vi "校准中 (子VI).vi"(0 "曲线模型":refnum<vi>, 1 "校准按钮":refnum<vi>) -> ()   [LabVIEW 2016, in "斯坦道氨氮.lvlib"]
uses:
  <vilib>/ptbypt/NI_PtbyPt.lvlib
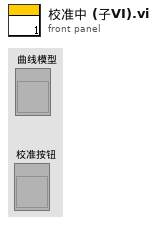
[diagram p1: front panel]
types:
  T1 = enum8{"Enabled", "Disabled", "Disabled and Grayed Out"}
  T2 = cluster{"时间标识":timestamp, "设备":string, "日志信息":string, "流程参数":string}
  T3 = cluster{"系统时间":timestamp, "工作状态":enum16{"空闲", "水样测试", "标样核查", "零点核查", "跨度核查", "空白测试", "平行样测试", "加标回收", "空白校准", "标样校准", "初始化（清洗）"}, "测量模式":enum16{"待机", "连续模式", "周期模式", "定点模式", "受控模式", "手动模式"}, "告警代码":u16, "故障代码":u16, "日志代码":u16, "软件版本":u16, "F0":sgl, "F1":sgl, "F2":sgl, "F3":sgl, "T":sgl, "H":sgl, "id":u16, "flowid":u16, "量程":u16, "总磷控温温度1":sgl, "营养盐控温温度2":sgl, "ADC":sgl}
  T4 = enum16{"空闲", "水样测试", "标样核查", "零点核查", "跨度核查", "空白测试", "平行样测试", "加标回收", "空白校准", "标样校准", "初始化（清洗）"}
  T5 = cluster{"因子编码":u32, "单位":u16, "标样参考值":sgl, "水样数据时间":timestamp, "水样实测值":sgl, "水样数据标识":string, "标样数据时间":timestamp, "标样实测值":sgl, "标样数据标识":string, "空白数据时间":timestamp, "空白实测值":sgl, "空白数据标识":string, "零点核查数据时间":timestamp, "零点核查实测值":sgl, "零点核查数据标识":string, "跨度核查数据时间":timestamp, "跨度核查实测值":sgl, "跨度核查数据标识":string, "加标回收数据时间":timestamp, "加标回收实测值":sgl, "加标回收数据标识":string, "平行样数据时间":timestamp, "平行样实测值":sgl, "平行样数据标识":string, "F0":sgl, "F1":sgl, "F2":sgl, "F3":sgl, "F4":sgl, "F5":sgl, "F6":sgl, "F7":sgl, "温度":sgl, "湿度":sgl, "X值":sgl, "fidrange":u16}
  T6 = cluster{"Value":dbl, "Value 2":dbl, "Value 3":dbl, "Value 4":dbl, "Value 5":dbl}
  T7 = cluster{"测量量程":dbl, "测量精度":dbl, "测量间隔":dbl, "消解温度":dbl, "消解时长":dbl, "空白校准时间":timestamp, "曲线截距":dbl, "曲线斜率":dbl, "测量检出限":dbl, "测量信号值":dbl, "线性相关系数":dbl, "二次多项式系数":dbl, "标样校准时间":timestamp, "稀释倍数":dbl, "三项式系数":dbl, "空白标定系数":dbl, "量程系数":dbl, "F0/ORPA":dbl, "F1/ORPB":dbl, "F2/ORPK":dbl, "F3":dbl, "F4":dbl, "F5":dbl, "F6":dbl, "F7":dbl, "X0/滴定数":dbl, "量程":dbl}
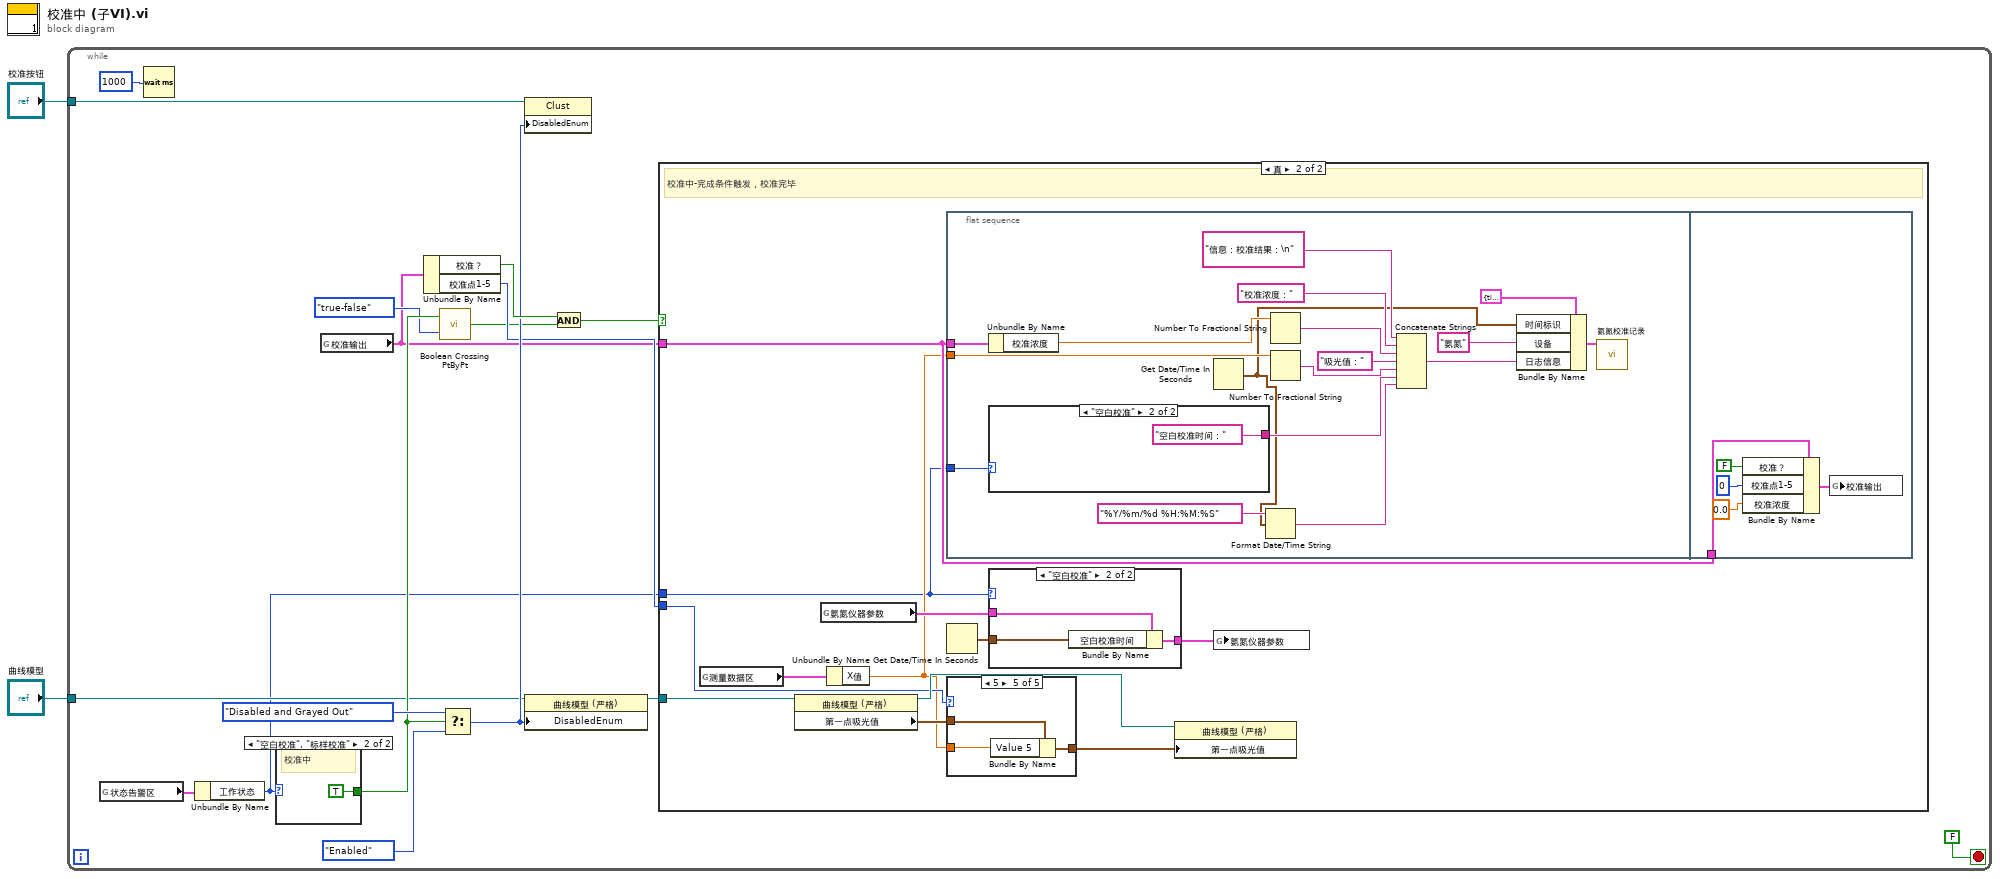
[diagram p0: block diagram]
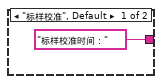
[diagram p3: hidden frame]
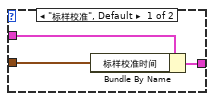
[diagram p4: hidden frame]
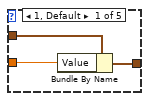
[diagram p5: hidden frame]
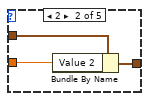
[diagram p6: hidden frame]
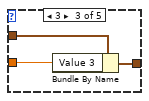
[diagram p7: hidden frame]
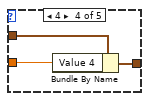
[diagram p8: hidden frame]
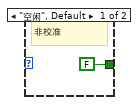
[diagram p9: hidden frame]
diagram:
  n1 = while {
    tunnel: "校准按钮" -> [w6]
    tunnel: "曲线模型" -> [w5]
    stop <- FALSE stop-if-true
    n2 = global read "VAR氨氮全局变量.vi" "状态告警区"() -> (w19:T3)
    n3 = Wait (ms)(milliseconds to wait=u32 1000 ("等待时间（毫秒）")) -> ()  [unwired: 1 out]
    n4 = Unbundle By Name(w19) -> ("工作状态"=w3:T4)
    n5 = case shown="\"空白校准\", \"标样校准\"" w3 {
      tunnel: [FALSE TRUE] -> w9
      frame "空闲", Default {
        # "非校准"
      }
      frame "空白校准", "标样校准" {
        # "校准中"
      }
    }
    n6 = global read "氨氮断电保存全局变量.vi" "校准输出"() -> (w4:cluster{"校准？":bool, "校准点1-5":u16, "校准浓度":dbl})
    n7 = Unbundle By Name(w4) -> ("校准？"=w18:bool, "校准点1-5"=w10:u16)
    n8 = call <vilib>:"Boolean Crossing PtByPt.vi"("direction"=enum16{"either", "false-true", "true-false"}."true-false", "input"=w9) -> ("crossing"=w7:bool)  [unwired: 1 in]
    n9 = Select(t=T1."Disabled and Grayed Out" ("禁用"), s=w9, f=T1."Enabled" ("禁用")) -> (s? t:f=w13:T1)
    n10 = property class="Clust"(reference=w6, "DisabledEnum"=w13) -> ()  [unwired: 1 in, 2 out]
    n11 = property class="曲线模型 (严格)"(reference=w5, "DisabledEnum"=w13) -> (reference out=w11:refnum<vi>)  [unwired: 1 in, 1 out]
    n12 = And(x=w18, y=w7) -> (x .and. y?=w12:bool)
    n13 = case shown="真" w12 {
      tunnel: w11 -> [_ w31]
      tunnel: w10 -> [_ w29]
      tunnel: w4 -> [_ w22]
      tunnel: w3 -> [_ w20]
      frame False {
      }
      frame True {
        # "校准中-完成条件触发，校准完毕"
        n14 = global read "VAR氨氮全局变量.vi" "测量数据区"() -> (w26:T5)
        n15 = property class="曲线模型 (严格)"(reference=w31) -> (reference out=w30:refnum<vi>, "第一点吸光值"=w28:T6)  [unwired: 1 in, 1 out]
        n16 = global read "氨氮断电保存全局变量.vi" "氨氮仪器参数"() -> (w25:T7)
        n17 = Unbundle By Name(w26) -> ("X值"=w21:sgl)
        n18 = flat-sequence {
          tunnel: w22 -> [w46]
          tunnel: w21 -> [w42]
          tunnel: w20 -> [w40]
          tunnel: w22 -> [w55]
          frame #0 {
            n19 = Unbundle By Name(w46) -> ("校准浓度"=w45:dbl)
            n20 = case shown="\"空白校准\"" w40 {
              tunnel: ["标样校准时间：" "空白校准时间："] -> w38
              frame "标样校准", Default {
              }
              frame "空白校准" {
              }
            }
            n21 = Get Date/Time In Seconds() -> (seconds since 1Jan1904=w35:timestamp)
            n22 = Format Date/Time String(time format string (%c)="%Y/%m/%d %H:%M:%S" ("时间格式字符串(%c)"), seconds (now)=w35) -> (date/time string=w37:string)  [unwired: 1 in]
            n23 = Number To Fractional String(number=w45) -> (F-format string=w44:string)  [unwired: 3 in]
            n24 = Number To Fractional String(number=w42) -> (F-format string=w41:string)  [unwired: 3 in]
            n25 = Concatenate Strings("信息：校准结果：\n", "校准浓度：", w44, "吸光值：", w41, w38, w37) -> (w33:string)
            n26 = Bundle By Name(cluster=T2 {"时间标识"=timestamp(0 s since 1904-01-01), "设备"="", "日志信息"="", "流程参数"=""} ("data in"), "时间标识"=w35, "设备"="氨氮", "日志信息"=w33) -> (w32:T2)
            n27 = call "氨氮校准记录.vi"("data in"=w32) -> ()  [unwired: 11 in]
          }
          frame #1 {
            n28 = Bundle By Name(cluster=w55, "校准？"=FALSE ("校准.校准？"), "校准点1-5"=u16 0 ("校准.校准点1-5"), "校准浓度"=0.0 ("校准.校准浓度")) -> (w51:cluster{"校准？":bool, "校准点1-5":u16, "校准浓度":dbl})
            n29 = global write "氨氮断电保存全局变量.vi" "校准输出"(w51) -> ()
          }
        }
        n30 = Get Date/Time In Seconds() -> (seconds since 1Jan1904=w23:timestamp)
        n31 = case shown="5" w29 {
          tunnel: w28 -> [w64 w67 w70 w73 w75]
          tunnel: [w63 w66 w69 w72 w76] -> w27
          tunnel: w21 -> [w62 w65 w68 w71 w74]
          frame 1, Default {
            n32 = Bundle By Name(cluster=w64, "Value"=w62) -> (w63:T6)
          }
          frame 2 {
            n33 = Bundle By Name(cluster=w67, "Value 2"=w65) -> (w66:T6)
          }
          frame 3 {
            n34 = Bundle By Name(cluster=w70, "Value 3"=w68) -> (w69:T6)
          }
          frame 4 {
            n35 = Bundle By Name(cluster=w73, "Value 4"=w71) -> (w72:T6)
          }
          frame 5 {
            n36 = Bundle By Name(cluster=w75, "Value 5"=w74) -> (w76:T6)
          }
        }
        n37 = case shown="\"空白校准\"" w20 {
          tunnel: w25 -> [w58 w60]
          tunnel: [w57 w59] -> w24
          tunnel: w23 -> [w56 w61]
          frame "标样校准", Default {
            n38 = Bundle By Name(cluster=w58, "标样校准时间"=w56) -> (w57:T7)
          }
          frame "空白校准" {
            n39 = Bundle By Name(cluster=w60, "空白校准时间"=w61) -> (w59:T7)
          }
        }
        n40 = property class="曲线模型 (严格)"(reference=w30, "第一点吸光值"=w27) -> ()  [unwired: 1 in, 2 out]
        n41 = global write "氨氮断电保存全局变量.vi" "氨氮仪器参数"(w24) -> ()
      }
    }
  }
